vi "Host_Automate_Full_Timing_Study.vi"() -> ()   [LabVIEW 2021]
panel:
  out "Elasped Time (h:m:s)":string caption="Result"
  out "Experiment progress":u8(slide) scale=0.0..300.0
  out "Current test":T1
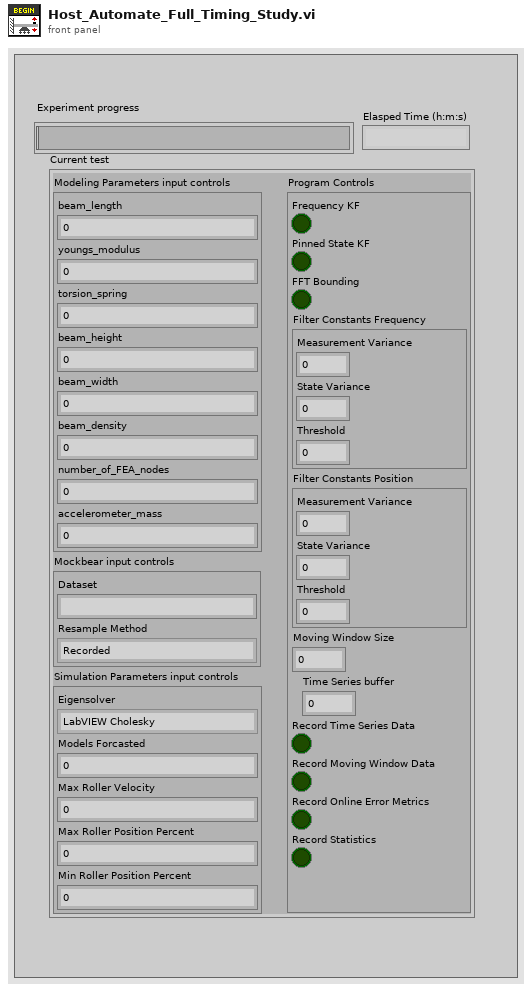
[diagram p1: front panel]
types:
  T1 = cluster{"Modeling Parameters input controls":cluster{"beam_length":dbl, "youngs_modulus":dbl, "torsion_spring":dbl, "beam_height":dbl, "beam_width":dbl, "beam_density":dbl, "number_of_FEA_nodes":i32, "accelerometer_mass":dbl}, "Mockbear input controls":cluster{"Dataset":string, "Resample Method":enum16{"Recorded", "Auto Resample", "Custom Resample"}}, "Simulation Parameters input controls":cluster{"Eigensolver ":enum16{"LabVIEW Cholesky", "LabVIEW General", "LabVIEW Inverse", "LEMP"}, "Models Forcasted":i32, "Max Roller Velocity":dbl, "Max Roller Position Percent":dbl, "Min Roller Position Percent":dbl}, "Program Controls":cluster{"Frequency KF":bool, "Pinned State KF":bool, "FFT Bounding":bool, "Filter Constants Frequency":cluster{"Measurement Variance":dbl, "State Variance":dbl, "Threshold":dbl}, "Filter Constants Position":cluster{"Measurement Variance":dbl, "State Variance":dbl, "Threshold":dbl}, "Moving Window Size":i32, "Time Series buffer":dbl, "Record Time Series Data":bool, "Record Moving Window Data":bool, "Record Online Error Metrics ":bool, "Record Statistics":bool}}
  T2 = cluster{"beam_length":dbl, "youngs_modulus":dbl, "torsion_spring":dbl, "beam_height":dbl, "beam_width":dbl, "beam_density":dbl, "number_of_FEA_nodes":i32, "accelerometer_mass":dbl}
  T3 = cluster{"Frequency KF":bool, "Pinned State KF":bool, "FFT Bounding":bool, "Filter Constants Frequency":cluster{"Measurement Variance":dbl, "State Variance":dbl, "Threshold":dbl}, "Filter Constants Position":cluster{"Measurement Variance":dbl, "State Variance":dbl, "Threshold":dbl}, "Moving Window Size":i32, "Time Series buffer":dbl, "Record Time Series Data":bool, "Record Moving Window Data":bool, "Record Online Error Metrics ":bool, "Record Statistics":bool}
  T4 = cluster{"Eigensolver ":enum16{"LabVIEW Cholesky", "LabVIEW General", "LabVIEW Inverse", "LEMP"}, "Models Forcasted":i32, "Max Roller Velocity":dbl, "Max Roller Position Percent":dbl, "Min Roller Position Percent":dbl}
  T5 = cluster{"Dataset":string, "Resample Method":enum16{"Recorded", "Auto Resample", "Custom Resample"}}
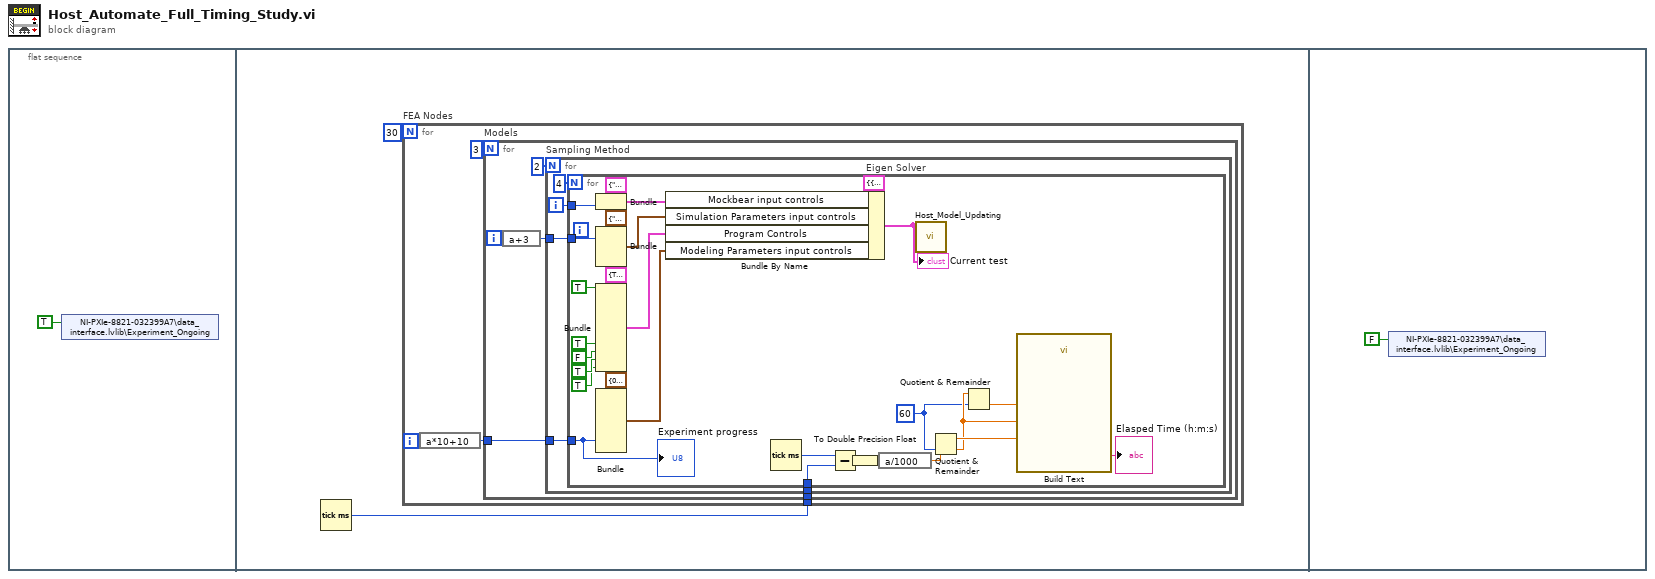
[diagram p0: block diagram]
diagram:
  n1 = flat-sequence {
    frame #0 {
      n2 = shared-variable "NI-PXIe-8821-032399A7\\data_interface.lvlib\\Experiment_Ongoing"(TRUE ("Experiment_Ongoing")) -> ()  [unwired: 1 in, 1 out]
    }
    frame #1 {
      n3 = Tick Count (ms)() -> (millisecond timer value=w2:u32)
      n4 = for "FEA Nodes" {
        N: 30 -> [_]
        tunnel: w2 -> [w4]
        i -> [w6]
        n5 = expression code="a*10+10"(w6) -> (w5:i32)
        n6 = for "Models" {
          N: 3 -> [_]
          tunnel: w5 -> [w9]
          tunnel: w4 -> [w8]
          i -> [w11]
          n7 = expression code="a+3"(w11) -> (w10:i32)
          n8 = for "Sampling Method" {
            N: 2 -> [_]
            tunnel: w10 -> [w15]
            tunnel: w9 -> [w14]
            tunnel: w8 -> [w13]
            i -> [w16]
            n9 = for "Eigen Solver" {
              N: 4 -> [_]
              tunnel: w16 -> [w37]
              tunnel: w15 -> [w36]
              tunnel: w14 -> [w28]
              tunnel: w13 -> [w27]
              w20 = 60
              n10 = Bundle(cluster=T5 {"Dataset"="test7", "Resample Method"=enum."Auto Resample"} ("Mockbear input controls"), "Resample Method"=w37) -> (w38:T5)  [unwired: 1 in]
              n11 = Bundle(cluster=T4 {"Eigensolver "=enum."LEMP", "Models Forcasted"=5, "Max Roller Velocity"=3.32, "Max Roller Position Percent"=0.43, "Min Roller Position Percent"=0.155} ("Simulation Parameters input controls"), "Models Forcasted"=w36) -> (w39:T4)  [unwired: 4 in]
              n12 = Bundle(cluster=T3 {"Frequency KF"=TRUE, "Pinned State KF"=FALSE, "FFT Bounding"=FALSE, "Filter Constants Frequency"={"Measurement Variance"=0.4, "State Variance"=0.01, "Threshold"=1000000000.0}, "Filter Constants Position"={"Measurement Variance"=0.4, "State Variance"=0.9, "Threshold"=1000000000.0}, "Moving Window Size"=10, "Time Series buffer"=10000.0, "Record Time Series Data"=FALSE, "Record Moving Window Data"=FALSE, "Record Online Error Metrics "=TRUE, "Record Statistics"=TRUE} ("Program Controls"), "Frequency KF"=TRUE, "Record Time Series Data"=TRUE, "Record Moving Window Data"=FALSE, "Record Online Error Metrics"=TRUE, "Record Statistics"=TRUE) -> (w44:T3)  [unwired: 6 in]
              n13 = Bundle(cluster=T2 {"beam_length"=0.3525, "youngs_modulus"=209500000000.0, "torsion_spring"=0.0, "beam_height"=0.00635, "beam_width"=0.0508, "beam_density"=7900.0, "number_of_FEA_nodes"=40, "accelerometer_mass"=0.055} ("Modeling Parameters input controls"), "number_of_FEA_nodes"=w28) -> (w34:T2)  [unwired: 7 in]
              n14 = Bundle By Name(cluster=T1 {"Modeling Parameters input controls"={"beam_length"=0.3525, "youngs_modulus"=209500000000.0, "torsion_spring"=0.0, "beam_height"=0.00635, "beam_width"=0.0508, "beam_density"=7900.0, "number_of_FEA_nodes"=40, "accelerometer_mass"=0.055}, "Mockbear input controls"={"Dataset"="test7", "Resample Method"=enum."Auto Resample"}, "Simulation Parameters input controls"={"Eigensolver "=enum."LEMP", "Models Forcasted"=5, "Max Roller Velocity"=3.32, "Max Roller Position Percent"=0.43, "Min Roller Position Percent"=0.155}, "Program Controls"={"Frequency KF"=TRUE, "Pinned State KF"=FALSE, "FFT Bounding"=FALSE, "Filter Constants Frequency"={"Measurement Variance"=0.4, "State Variance"=0.01, "Threshold"=1000000000.0}, "Filter Constants Position"={"Measurement Variance"=0.4, "State Variance"=0.9, "Threshold"=1000000000.0}, "Moving Window Size"=10, "Time Series buffer"=10000.0, "Record Time Series Data"=FALSE, "Record Moving Window Data"=FALSE, "Record Online Error Metrics "=TRUE, "Record Statistics"=TRUE}} ("Setup Parameters and Controls"), "Mockbear input controls"=w38, "Simulation Parameters input controls"=w39, "Program Controls"=w44, "Modeling Parameters input controls"=w34) -> (w45:T1)
              "Current test" <- w45
              n15 = Tick Count (ms)() -> (millisecond timer value=w26:u32)
              n16 = Subtract(x=w26, y=w27) -> (x-y=w25:u32)
              n17 = To Double Precision Float(number=w25) -> (double precision float=w19:dbl)
              n18 = expression code="a/1000"(w19) -> (w22:dbl)
              n19 = call "Host_Model_Updating.vi"("Setup Parameters and Controls"=w45) -> ()  [unwired: 11 in]
              n20 = Quotient & Remainder(x=w22, y=w20) -> (x-y*floor(x/y)=w23:dbl, floor(x/y)=w21:dbl)
              n21 = Quotient & Remainder(x=w21, y=w20) -> (floor(x/y)=w24:dbl)  [unwired: 1 out]
              n22 = call "Build Text"("hours"=w24, "minutes"=w21, "seconds"=w23) -> ("Result"=→"Elasped Time (h:m:s)":string)  [unwired: 11 in, 1 out]
              "Experiment progress" <- w28
            }
          }
        }
      }
    }
    frame #2 {
      n23 = shared-variable "NI-PXIe-8821-032399A7\\data_interface.lvlib\\Experiment_Ongoing"(FALSE ("Experiment_Ongoing")) -> ()  [unwired: 1 in, 1 out]
    }
  }
